vi "GetSelectedChannelProperties.vi"(8 "error in (no error)":errorcluster, 11 "Highland T564 DDG in":refnum<class "Highland T564 DDG.lvclass">) -> (0 "error out":errorcluster, 3 "ChannelProperties":variant)   [LabVIEW 2020, in "Highland T564 DDG.lvclass"]
uses:
  Highland T564 DDG.lvclass
  C:/GEECS/Developers Version/source/Device Drivers/shared/MetaDriver_v1/MetaDriver_v1.lvclass
  Highland T564 DDG.lvclass/Highland T564 DDG.ctl
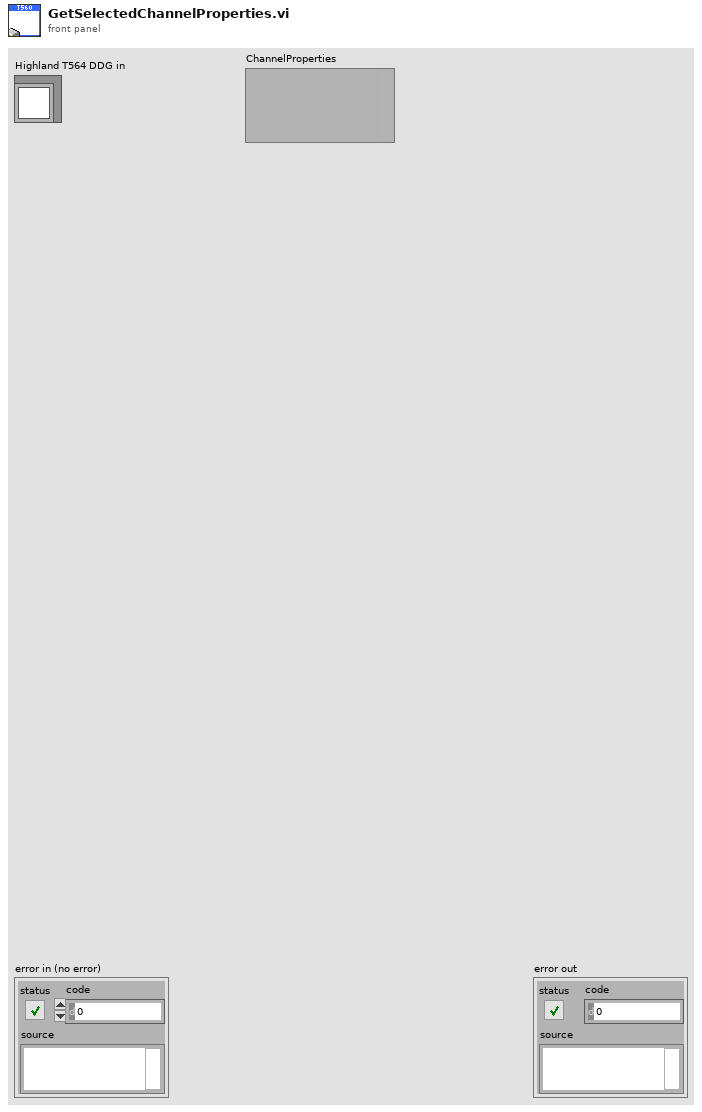
[diagram p1: front panel]
types:
  T1 = typedef "Highland T564 DDG.lvclass/settings Highland T560 DDG_TypDef.ctl" = cluster{"VisaResource":string, "BaudRate":u32, "Save":enum16{"off", "on"}, "LocalSavingPath":path, "Trigger":T2, "Channel1":T6, "Channel2":T6, "Channel3":T6, "Channel4":T6, "Simulation":T9}
  T2 = typedef "Trigger.ctl" = cluster{"Divisor":T3, "Level":T3, "Impedance":T4, "Source":T5}
  T3 = typedef "Choice01.ctl" = cluster{"Value":dbl, "Min":dbl, "Max":dbl, "StepSize":dbl, "Tolerance":dbl, "ValueActual":dbl}
  T4 = typedef "TriggerImpedance.ctl" = enum16{"10KOhm", "50Ohms"}
  T5 = typedef "TriggerSource.ctl" = enum16{"Rising", "Falling", "Internal 80MHz", "Internal DDS", "Remote", "Disabled"}
  T6 = typedef "Channel.ctl" = cluster{"Polarity":T7, "ChannelOn":enum16{"off", "on"}, "Delay":T3, "Width":T3, "ChannelName":T8}
  T7 = typedef "Choice83.ctl" = enum16{"Direct", "Inverted"}
  T8 = typedef "Choice84.ctl" = enum16{"Null", "A", "B", "C", "D", "Trigger"}
  T9 = typedef "OnOffTypeDef.ctl" = enum16{"off", "on"}
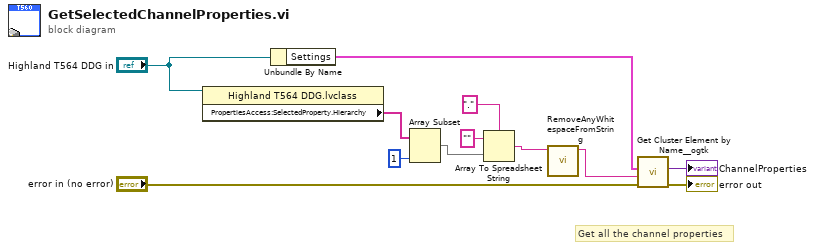
[diagram p0: block diagram]
diagram:
  # "Get all the channel properties"
  n1 = property class="Highland T564 DDG.lvclass"(reference="Highland T564 DDG in") -> ("PropertiesAccess:SelectedProperty.Hierarchy"=w1:string[])  [unwired: 1 in, 2 out]
  n2 = Unbundle By Name("Highland T564 DDG in") -> ("Settings"=w3:T1)
  n3 = Array Subset(array=w1, length=1) -> (w9:string[])  [unwired: 1 in]
  n4 = Array To Spreadsheet String(delimiter (Tab)=".", array=w9, 3:"" ("format string")) -> (spreadsheet string=w11:string)
  n5 = call "RemoveAnyWhitespaceFromString.vi"("String in"=w11) -> ("String out"=w12:string)  [unwired: 10 in]
  n6 = call <userlib>:"Get Cluster Element by Name__ogtk.vi"("error in (no error)"="error in (no error)", "Element Name"=w12, "Cluster"=w3) -> ("error out"=→"error out":errorcluster, "VElement"=→"ChannelProperties":variant)  [unwired: 6 in, 1 out]
